vi "CsTool-CaptureFill.vi"(1 "Handle Cluster":T1) -> (0 "Error Code":i32)   [LabVIEW 2022 SP3]
doc: "Calling this VI starts an acquisition by the CompuScope system identified by Handle Cluster, which is obtained by using CsTool-GetSystem.vi. The CompuScope system will start digitizing pre-trigger data into on-board memory until a trigger event occurs. Once the trigger event occurs, the specified number of post-trigger points will be captured and then the acquisition will terminate.\n\nIf the call is successful, a 1 is returned in the Error Code indicator. Otherwise, an error code is returned. A descriptive error string may be obtained by using CsTool-ErrorHandler.vi."
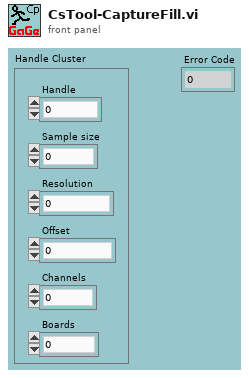
[diagram p1: front panel]
types:
  T1 = cluster{"Handle":u32, "Sample size":u32, "Resolution":i32, "Offset":i32, "Channels":u32, "Boards":u32}
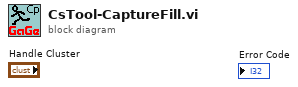
[diagram p0: block diagram]
diagram:
